vi "PH_Beckhoff_10BB_Plus.panel.vi"(0 "object ref":refnum<vi>, 5 "error in (no error)":errorcluster) -> (19 "error out":errorcluster)   [LabVIEW 2014, in "PH_Beckhoff_10BB_Plus.lvlib"]
doc: "This a GUI.\n\nLicense Agreement for this software:\n\nCopyright (C)\nGesellschaft für Schwerionenforschung, GSI\nPlanckstr. 1\n64291 Darmstadt\nGermany\n\nContact: D.Beck@gsi.de \n\nThis program is free software; you can redistribute it and/or modify it under the terms of the GNU General Public License as published by the Free Software Foundation; either version 2 of the license, or (at your option) any later version.\n\nThis program is distributed in the hope that it will be useful, but WITHOUT ANYW ARRANTY; without even the implied warranty of MERCHANTABILITY or FITNESS FOR A PARTICULAR PURPOSE. See the GNU General License for more details (http://www.gnu.org).\n\nGesellschaft für Schwerionenforschung, GSI\nPlanckstr. 1, 64291 Darmstadt, Germany\nFor all questions and ideas contact: M.Richter@gsi.de, H.Brand@gsi.de or D.Beck@gsi.de.\nLast update: 18-DEC-2002"
uses:
  PH_Beckhoff_10BB_Plus.lvlib
  PH_Beckhoff/PH_Beckhoff.Connectivity.ctl
  PH_Beckhoff/PH_Beckhoff.Values.ctl
  PH_Beckhoff/PH_Beckhoff.Sonderklemmen Inputs.ctl
  PH_Beckhoff/PH_Beckhoff.Analog Inputs.ctl
  PH_Beckhoff/PH_Beckhoff.Scaling Type.ctl
  PH_Beckhoff/PH_Beckhoff.Analog Outputs.ctl
  PH_Beckhoff/PH_Beckhoff.Digital Inputs.ctl
  PH_Beckhoff/PH_Beckhoff.Digital Outputs.ctl
  PH_Beckhoff/PH_Beckhoff.ADS Error.ctl
  PH_Beckhoff/PH_Beckhoff.GUI Refs.ctl
  CSCore/CSObj/CSObj.lvlib
  PH_Common/PH_Common.lvlib
  PH_Beckhoff/PH_Beckhoff.lvlib
  CSCore/CSSystem/CSSystemLib/CSSystemLib.lvlib
  PH_Class/PH_Class.lvlib
panel:
  out "configured?":bool
  out "ADS Error":T1
  in  "Show Info":bool
  out "Values":T2
  out "Prdc Int [ms]":i32
  out "Connection":T9
  out "IP":string
  in  "Delete":bool
  in  "Exit":bool
  # "PCS"
  # "3.40"
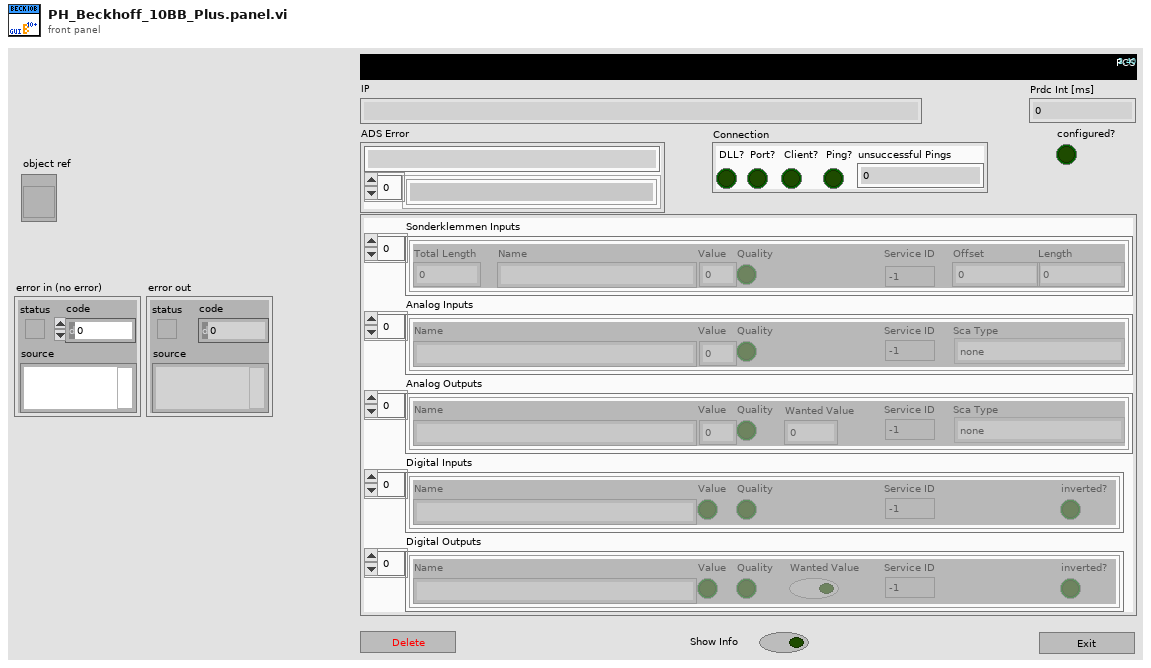
[diagram p1: front panel]
types:
  T1 = typedef "PH_Beckhoff.lvlib/PH_Beckhoff.ADS Error.ctl" = cluster{"Latest Error":string, "Error List":string[]}
  T2 = typedef "PH_Beckhoff.lvlib/PH_Beckhoff.Values.ctl" = cluster{"Sonderklemmen Inputs":T3, "Analog Inputs":T4, "Analog Outputs":T6, "Digital Inputs":T7, "Digital Outputs":T8}
  T3 = typedef "PH_Beckhoff.lvlib/PH_Beckhoff.Sonderklemmen Inputs.ctl" = cluster{"Total Length":u32, "Name":string, "Value":u64, "Quality":bool, "Service ID":i32, "Offset":u32, "Length":u32}[]
  T4 = typedef "PH_Beckhoff.lvlib/PH_Beckhoff.Analog Inputs.ctl" = cluster{"Name":string, "Value":u32, "Quality":bool, "Service ID":i32, "Sca Type":T5}[]
  T5 = typedef "PH_Beckhoff.lvlib/PH_Beckhoff.Scaling Type.ctl" = enum16{"none", "0 ... 15 Bit -> 0 ... 5", "0 ... 15 Bit -> 0 ... 10", "0 ... 15 Bit -> 0 ... 25", "0 ... 15 Bit -> 4 ... 20", "0 ... 15 Bit -> 0 ... 1", "0 ... 15 Bit -> 0 ... 20000", "0 ... 15 Bit -> 0 ... 24000"}
  T6 = typedef "PH_Beckhoff.lvlib/PH_Beckhoff.Analog Outputs.ctl" = cluster{"Name":string, "Value":u32, "Quality":bool, "Wanted Value":u32, "Service ID":i32, "Sca Type":T5}[]
  T7 = typedef "PH_Beckhoff.lvlib/PH_Beckhoff.Digital Inputs.ctl" = cluster{"Name":string, "Value":bool, "Quality":bool, "Service ID":i32, "inverted?":bool}[]
  T8 = typedef "PH_Beckhoff.lvlib/PH_Beckhoff.Digital Outputs.ctl" = cluster{"Name":string, "Value":bool, "Quality":bool, "Wanted Value":bool, "Service ID":i32, "inverted?":bool}[]
  T9 = typedef "PH_Beckhoff.lvlib/PH_Beckhoff.Connectivity.ctl" = cluster{"DLL?":bool, "Port?":bool, "Client?":bool, "Ping?":bool, "unsuccessful Pings":u32}
  T10 = typedef "PH_Beckhoff.lvlib/PH_Beckhoff.GUI Refs.ctl" = cluster{"ADS Error":refnum<vi>, "Values":refnum<vi>, "configured?":refnum<vi>, "Connection":refnum<vi>, "IP":refnum<vi>, "Prdc Int [ms]":refnum<vi>}
  T11 = typedef "PH_Beckhoff.lvlib/PH_Beckhoff.i attribute.ctl" = cluster{"GUI Refs":T10, "operation?":bool, "Default Prdc Interval":i32, "Connection":T9, "AMS Net ID":T12, "Klemmencluster: # of":T13, "Values":T2, "IP":string, "Description":string, "configured?":bool, "Change Manager":cluster{"Detemination wanted?":bool, "Values changed at":cluster{"Sonderklemmen Inputs":i32[], "Analog Inputs":i32[], "Analog Outputs":i32[], "Digital Inputs":i32[], "Digital Outputs":i32[]}}, "Difference to handle an analog input as change":u32}
  T12 = typedef "Beckhoff - Driver np.lvlib/Beckhoff Access.ctl" = cluster{"DLL path":path, "AMS Net ID":cluster{"1st # of IP":u8, "2nd # of IP":u8, "3rd # of IP":u8, "4th # of IP":u8, "In Port":u8, "Out Port":u8}}
  T13 = typedef "Beckhoff - Driver np.lvlib/Klemmendeclarer.ctl" = cluster{"Offset due to Sonderklemms":u32, "analog Inputs":u32, "analog Outputs":u32, "digital Input Bits":u32, "digital Output Bits":u32}
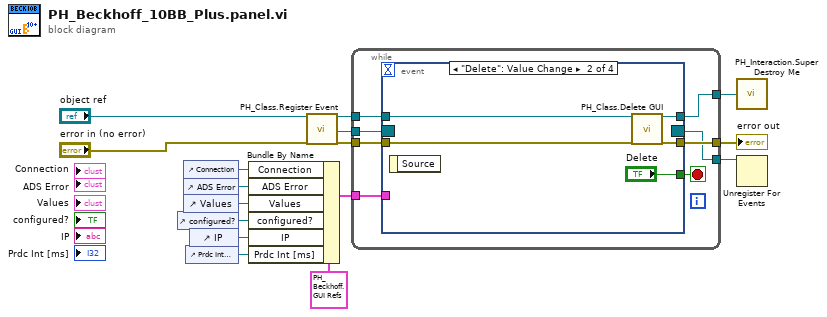
[diagram p0: block diagram]
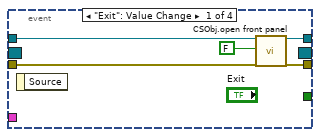
[diagram p2: hidden frame]
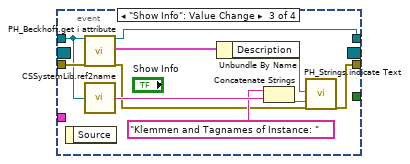
[diagram p3: hidden frame]
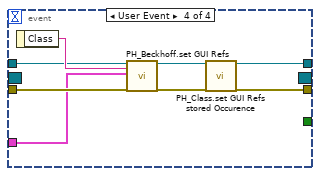
[diagram p4: hidden frame]
diagram:
  n1 = control-ref of="configured?"() -> (w10:refnum<vi>)
  n2 = control-ref of="Connection"() -> (w14:refnum<vi>)
  n3 = control-ref of="ADS Error"() -> (w12:refnum<vi>)
  n4 = control-ref of="Values"() -> (w13:refnum<vi>)
  n5 = control-ref of="Prdc Int [ms]"() -> (w1:refnum<vi>)
  n6 = control-ref of="IP"() -> (w2:refnum<vi>)
  n7 = Bundle By Name(cluster=T10 {"ADS Error"=refnum, "Values"=refnum, "configured?"=refnum, "Connection"=refnum, "IP"=refnum, "Prdc Int [ms]"=refnum} ("GUI Refs"), "Connection"=w14, "ADS Error"=w12, "Values"=w13, "configured?"=w10, "IP"=w2, "Prdc Int [ms]"=w1) -> (w6:T10)
  n8 = call "PH_Class.Register Event.vi"("i ref in"="object ref", "error in (no error)"="error in (no error)") -> ("i ref out"=w9:refnum<vi>, "Event Registration Refnum"=w7:refnum<event-registration>, "error out"=w8:errorcluster)  [unwired: 15 in]
  n9 = while {
    tunnel: w9 -> [w21]
    tunnel: [w20] -> w16
    tunnel: w8 -> [w23]
    tunnel: [w22] -> w15
    tunnel: w7 -> [w19]
    tunnel: w6 -> [w18]
    tunnel: [w17] -> w5
    stop <- w24 stop-if-true
    n10 = event shown="[1] \"Delete\": Value Change" {
      selector: w19 -> [_ _ _ _]
      dyn-events: [_ _ _ _] -> w17
      timeout: _ -> [_ _ _ _]
      tunnel: [_ "Delete" _ _] -> w24
      tunnel: w21 -> [w26 w31 w35 w51]
      tunnel: w23 -> [w29 w33 w38 w50]
      tunnel: [w28 w32 w36 w47] -> w22
      tunnel: [w25 w30 w37 w45] -> w20
      tunnel: w18 -> [_ _ _ w48]
      event "Exit": Value Change {
        n11 = event-data() -> ()  [unwired: 1 in, 1 out]
        n12 = call "CSObj.open front panel.vi"("i ref in"=w26, "frontPanelOpen"=FALSE ("front panel open"), "error in (no error)"=w29) -> ("i ref out"=w25:refnum<vi>, "error out"=w28:errorcluster)  [unwired: 15 in]
      }
      event "Delete": Value Change {
        n13 = event-data() -> ()  [unwired: 1 in, 1 out]
        n14 = call "PH_Class.Delete GUI.vi"("VI in"=w31, "error in (no error)"=w33) -> ("VI out"=w30:refnum<vi>, "error out"=w32:errorcluster)  [unwired: 16 in]
      }
      event "Show Info": Value Change {
        n15 = event-data() -> ()  [unwired: 1 in, 1 out]
        n16 = call "PH_Beckhoff.get i attribute.vi"("i ref in"=w35, "error in (no error)"=w38) -> ("i ref out"=w37:refnum<vi>, "i attribute"=w40:T11, "error out"=w39:errorcluster)  [unwired: 15 in]
        n17 = call "CSSystemLib.ref2name.vi"("obj refnum"=w35) -> ("name"=w44:string)
        n18 = Unbundle By Name(w40) -> ("Description"=w41:string)
        n19 = Concatenate Strings("Klemmen and Tagnames of Instance: " ("Caption.Text"), w44) -> (w43:string)
        n20 = call "PH_Strings.indicate Text.vi"("String to show"=w41, "Caption.Text"=w43, "error in (no error)"=w39) -> ("error out"=w36:errorcluster)  [unwired: 16 in]
      }
      event User Event {
        n21 = event-data() -> ("Class"=w52:string)  [unwired: 1 in]
        n22 = call "PH_Beckhoff.set GUI Refs.vi"("i ref in"=w51, "Class"=w52, "GUI Refs"=w48, "error in"=w50) -> ("i ref out"=w46:refnum<vi>, "error out"=w49:errorcluster)  [unwired: 14 in]
        n23 = call "PH_Class.set GUI Refs stored Occurence.vi"("i ref in"=w46, "error in (no error)"=w49) -> ("i ref out"=w45:refnum<vi>, "error out"=w47:errorcluster)  [unwired: 16 in]
      }
    }
  }
  "error out" <- w15
  n24 = call "PH_Interaction.Super Destroy Me.vi"("i ref out"=w16) -> ()
  n25 = Unregister For Events(event registration refnum=w5) -> ()  [unwired: 1 in, 1 out]
